vi "rapid.vi"(0 "Speed":refnum<vi>, 1 "positon":refnum<vi>, 2 "Reverse":refnum<vi>, 3 "Power":refnum<vi>, 4 "Rapid":refnum<vi>, 5 "Set x":dbl min=0.0, 6 "Input":dbl, 7 "Zero":refnum<vi>) -> ()   [LabVIEW 2017]
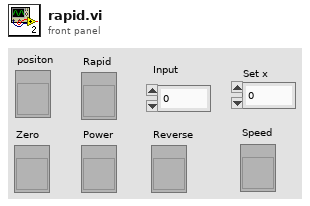
[diagram p1: front panel]
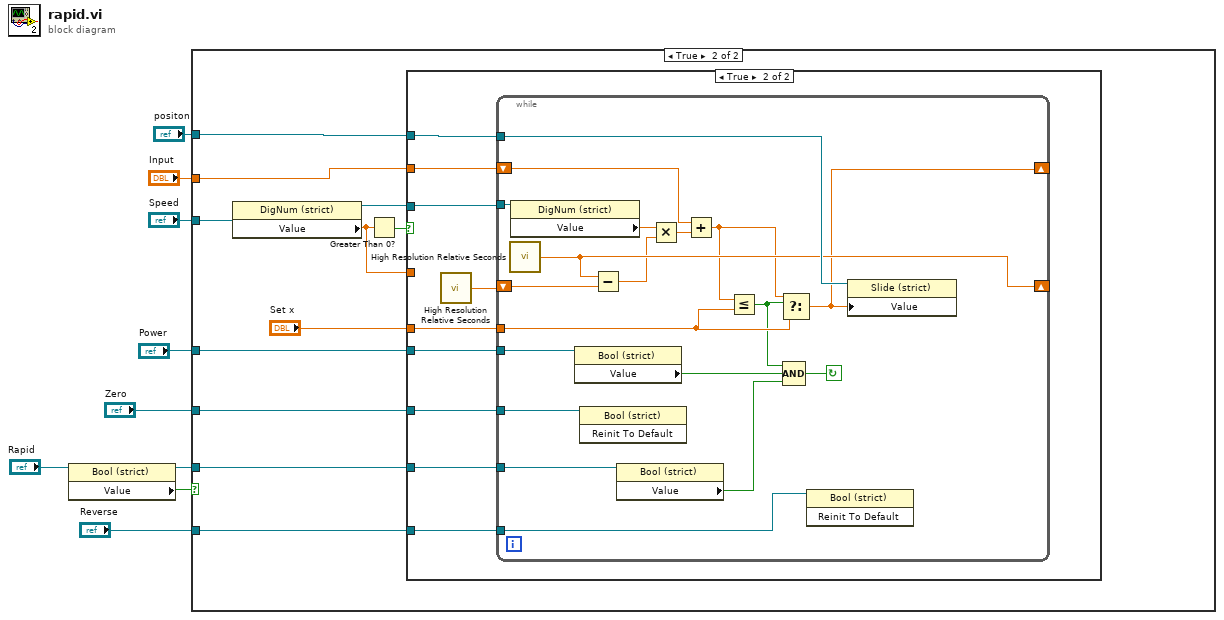
[diagram p0: block diagram]
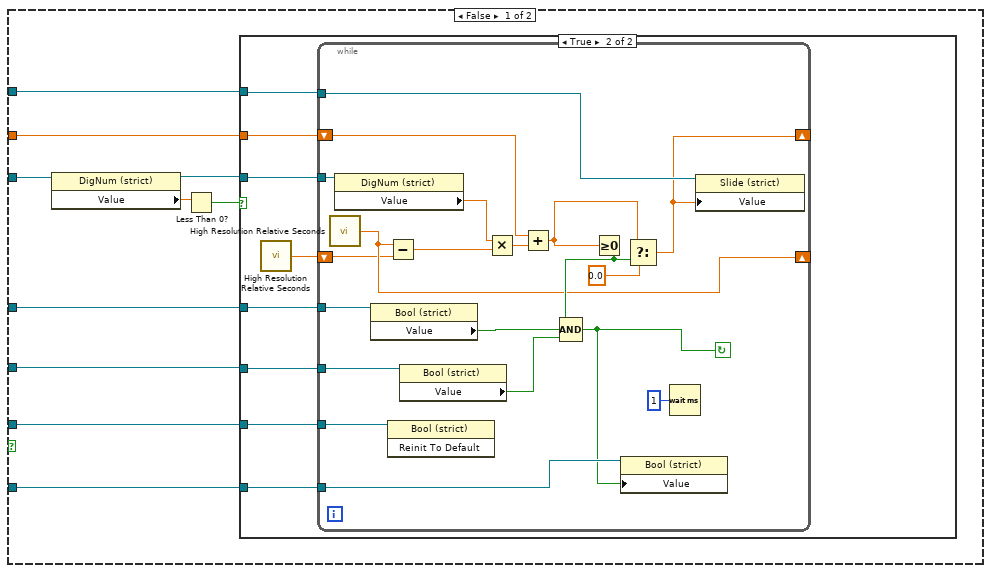
[diagram p2: hidden frame]
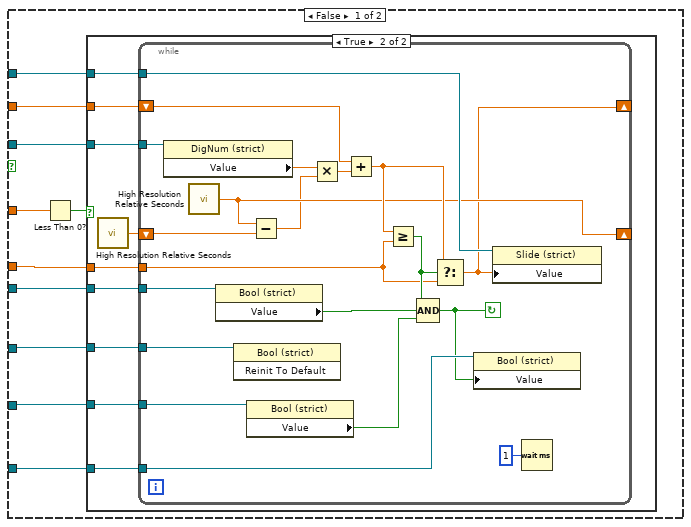
[diagram p4: hidden frame]
diagram:
  n1 = property class="Bool (strict)"(reference="Rapid") -> (reference out=w4:refnum<vi>, "Value"=w6:bool)  [unwired: 1 in, 1 out]
  n2 = case shown="True" w6 {
    tunnel: "Input" -> [w19 w58]
    tunnel: "positon" -> [w18 w57]
    tunnel: "Zero" -> [w10 w53]
    tunnel: w4 -> [w17 w55]
    tunnel: "Power" -> [w16 w54]
    tunnel: "Reverse" -> [w15 w52]
    tunnel: "Speed" -> [w14 w51]
    frame False {
      n3 = property class="DigNum (strict)"(reference=w14) -> (reference out=w12:refnum<vi>, "Value"=w13:dbl)  [unwired: 1 in, 1 out]
      n4 = Less Than 0?(x=w13) -> (x < 0?=w11:bool)
      n5 = case shown="True" w11 {
        tunnel: w19 -> [_ w27]
        tunnel: w18 -> [_ w26]
        tunnel: w10 -> [_ w25]
        tunnel: w17 -> [_ w24]
        tunnel: w16 -> [_ w23]
        tunnel: w15 -> [_ w22]
        tunnel: w12 -> [_ w21]
        frame False {
        }
        frame True {
          n6 = call <vilib>:"High Resolution Relative Seconds.vi"() -> ("relative seconds"=w20:dbl)
          n7 = while {
            tunnel: w26 -> [w43]
            tunnel: w25 -> [w42]
            tunnel: w24 -> [w39]
            tunnel: w23 -> [w41]
            tunnel: w22 -> [w37]
            shift-right: [w35] -> _
            shift-left: w20 -> [w31]
            tunnel: w21 -> [w33]
            shift-right: [w29] -> _
            shift-left: w27 -> [w47]
            stop <- w36 continue-if-true
            n8 = call <vilib>:"High Resolution Relative Seconds.vi"() -> ("relative seconds"=w35:dbl)
            n9 = property class="DigNum (strict)"(reference=w33) -> ("Value"=w32:dbl)  [unwired: 1 in, 2 out]
            n10 = property class="Bool (strict)"(reference=w41) -> ("Value"=w40:bool)  [unwired: 1 in, 2 out]
            n11 = Subtract(x=w35, y=w31) -> (x-y=w34:dbl)
            n12 = invoke class="Bool (strict)" method="Reinit To Default"(reference=w39) -> ()  [unwired: 2 in, 3 out]
            n13 = property class="Bool (strict)"(reference=w42) -> ("Value"=w38:bool)  [unwired: 1 in, 2 out]
            n14 = Multiply(x=w32, y=w34) -> (x*y=w30:dbl)
            n15 = Add(x=w47, y=w30) -> (x+y=w46:dbl)
            n16 = Greater Or Equal To 0?(x=w46) -> (x >= 0?=w44:bool)
            n17 = Compound Arithmetic op=AND(w44, w40, w38) -> (w36:bool)
            n18 = property class="Bool (strict)"(reference=w37, "Value"=w36) -> ()  [unwired: 1 in, 2 out]
            n19 = Select(t=w46, s=w44, f=0.0) -> (s? t:f=w29:dbl)
            n20 = Wait (ms)(milliseconds to wait=u32 1) -> ()  [unwired: 1 out]
            n21 = property class="Slide (strict)"(reference=w43, "Value"=w29) -> ()  [unwired: 1 in, 2 out]
          }
        }
      }
    }
    frame True {
      n22 = property class="DigNum (strict)"(reference=w51) -> (reference out=w50:refnum<vi>, "Value"=w48:dbl)  [unwired: 1 in, 1 out]
      n23 = Greater Than 0?(x=w48) -> (x > 0?=w49:bool)
      n24 = case shown="True" w49 {
        tunnel: "Set x" -> [w67 w106]
        tunnel: w58 -> [w65 w105]
        tunnel: w57 -> [w66 w104]
        tunnel: w55 -> [w64 w103]
        tunnel: w54 -> [w63 w102]
        tunnel: w53 -> [w62 w101]
        tunnel: w52 -> [w61 w100]
        tunnel: w50 -> [w60 w98]
        tunnel: w48 -> [w59 _]
        frame False {
          n25 = Less Than 0?(x=w59) -> (x < 0?=w68:bool)
          n26 = case shown="True" w68 {
            tunnel: w67 -> [_ w76]
            tunnel: w66 -> [_ w75]
            tunnel: w65 -> [_ w77]
            tunnel: w64 -> [_ w74]
            tunnel: w63 -> [_ w73]
            tunnel: w62 -> [_ w72]
            tunnel: w61 -> [_ w71]
            tunnel: w60 -> [_ w69]
            frame False {
            }
            frame True {
              n27 = call <vilib>:"High Resolution Relative Seconds.vi"() -> ("relative seconds"=w70:dbl)
              n28 = while {
                tunnel: w76 -> [w92]
                tunnel: w75 -> [w95]
                tunnel: w74 -> [w93]
                tunnel: w73 -> [w91]
                tunnel: w72 -> [w88]
                tunnel: w71 -> [w87]
                shift-right: [w84] -> _
                shift-left: w70 -> [w85]
                tunnel: w69 -> [w83]
                shift-right: [w79] -> _
                shift-left: w77 -> [w97]
                stop <- w86 continue-if-true
                n29 = property class="DigNum (strict)"(reference=w83) -> ("Value"=w82:dbl)  [unwired: 1 in, 2 out]
                n30 = call <vilib>:"High Resolution Relative Seconds.vi"() -> ("relative seconds"=w84:dbl)
                n31 = property class="Bool (strict)"(reference=w91) -> ("Value"=w90:bool)  [unwired: 1 in, 2 out]
                n32 = invoke class="Bool (strict)" method="Reinit To Default"(reference=w88) -> ()  [unwired: 2 in, 3 out]
                n33 = property class="Bool (strict)"(reference=w93) -> ("Value"=w89:bool)  [unwired: 1 in, 2 out]
                n34 = Subtract(x=w84, y=w85) -> (x-y=w81:dbl)
                n35 = Multiply(x=w82, y=w81) -> (x*y=w80:dbl)
                n36 = Add(x=w97, y=w80) -> (x+y=w96:dbl)
                n37 = Greater Or Equal?(x=w96, y=w92) -> (x >= y?=w94:bool)
                n38 = Compound Arithmetic op=AND(w94, w90, w89) -> (w86:bool)
                n39 = Select(t=w96, s=w94, f=w92) -> (s? t:f=w79:dbl)
                n40 = property class="Bool (strict)"(reference=w87, "Value"=w86) -> ()  [unwired: 1 in, 2 out]
                n41 = property class="Slide (strict)"(reference=w95, "Value"=w79) -> ()  [unwired: 1 in, 2 out]
                n42 = Wait (ms)(milliseconds to wait=u32 1) -> ()  [unwired: 1 out]
              }
            }
          }
        }
        frame True {
          n43 = call <vilib>:"High Resolution Relative Seconds.vi"() -> ("relative seconds"=w99:dbl)
          n44 = while {
            tunnel: w106 -> [w108]
            tunnel: w104 -> [w124]
            tunnel: w103 -> [w123]
            tunnel: w102 -> [w121]
            tunnel: w101 -> [w119]
            tunnel: w100 -> [w118]
            shift-right: [w116] -> _
            shift-left: w99 -> [w117]
            tunnel: w98 -> [w115]
            shift-right: [w111] -> _
            shift-left: w105 -> [w112]
            stop <- w125 continue-if-true
            n45 = call <vilib>:"High Resolution Relative Seconds.vi"() -> ("relative seconds"=w116:dbl)
            n46 = property class="DigNum (strict)"(reference=w115) -> ("Value"=w110:dbl)  [unwired: 1 in, 2 out]
            n47 = property class="Bool (strict)"(reference=w121) -> ("Value"=w120:bool)  [unwired: 1 in, 2 out]
            n48 = invoke class="Bool (strict)" method="Reinit To Default"(reference=w119) -> ()  [unwired: 2 in, 3 out]
            n49 = Subtract(x=w116, y=w117) -> (x-y=w114:dbl)
            n50 = property class="Bool (strict)"(reference=w123) -> ("Value"=w122:bool)  [unwired: 1 in, 2 out]
            n51 = Multiply(x=w110, y=w114) -> (x*y=w113:dbl)
            n52 = Add(x=w112, y=w113) -> (x+y=w109:dbl)
            n53 = Less Or Equal?(x=w109, y=w108) -> (x <= y?=w107:bool)
            n54 = Select(t=w109, s=w107, f=w108) -> (s? t:f=w111:dbl)
            n55 = Compound Arithmetic op=AND(w107, w120, w122) -> (w125:bool)
            n56 = invoke class="Bool (strict)" method="Reinit To Default"(reference=w118) -> ()  [unwired: 2 in, 3 out]
            n57 = property class="Slide (strict)"(reference=w124, "Value"=w111) -> ()  [unwired: 1 in, 2 out]
          }
        }
      }
    }
  }
